vi "Create Field.vi"(8 "Field ID Counter":i32, 10 "Variant":variant, 11 "Field Name":string) -> (0 "Found":bool, 1 "Field ID":i32, 3 "Variant out":variant)   [LabVIEW 2017]
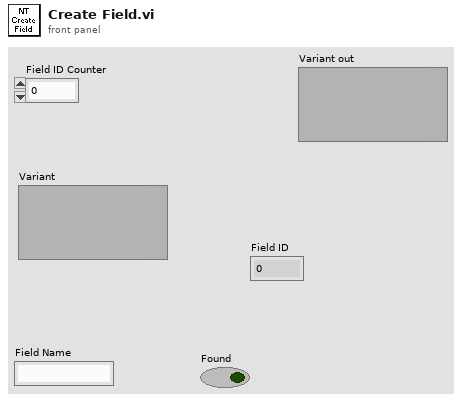
[diagram p1: front panel]
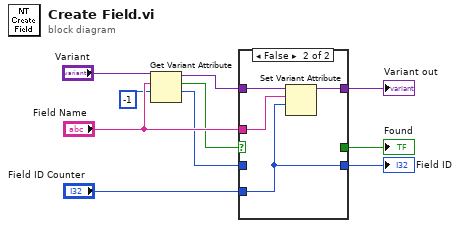
[diagram p0: block diagram]
diagram:
  n1 = Get Variant Attribute(Variant="Variant", name="Field Name", default value (empty Variant)=-1) -> (duplicate Variant=w1:variant, found=w4:bool, value=w3:i32)  [unwired: 1 in, 1 out]
  n2 = case shown="False" w4 {
    selector: w4 -> [w11 _]
    tunnel: w1 -> [w13 w15]
    tunnel: [w13 w14] -> w7
    tunnel: "Field Name" -> [_ w17]
    tunnel: [w11 _] -> w8
    tunnel: "Field ID Counter" -> [_ w16]
    tunnel: [w12 w16] -> w6
    tunnel: w3 -> [w12 _]
    frame True {
      # "Already present"
    }
    frame False {
      n3 = Set Variant Attribute(Variant=w15, name=w17, value=w16) -> (Variant out=w14:variant)  [unwired: 1 in, 2 out]
    }
  }
  "Found" <- w8
  "Variant out" <- w7
  "Field ID" <- w6
